vi "Biometry Average PD Parameter2String.vi"(8 "error in (no error)":errorcluster caption="错误输入（无错误）", 9 "Biometry Average Standard Deviation":T1, 10 "Biometry Average State":T2, 11 "Biometry Average Parameter":T3) -> (0 "error out":errorcluster caption="错误输出", 2 "Data Output":string[][](array[string]))   [LabVIEW 2015, in "Utility VIs.lvlib"]
doc: "该模板用于创建子VI。"
uses:
  Utility VIs.lvlib
  Database Processing/Support/Table/Biometry Average Parameter.ctl
  Database Processing/Support/Table/Biometry Average State.ctl
  Database Processing/Support/Table/Biometry Average Standard Deviation.ctl
  Database Processing/Database Processing.lvlib
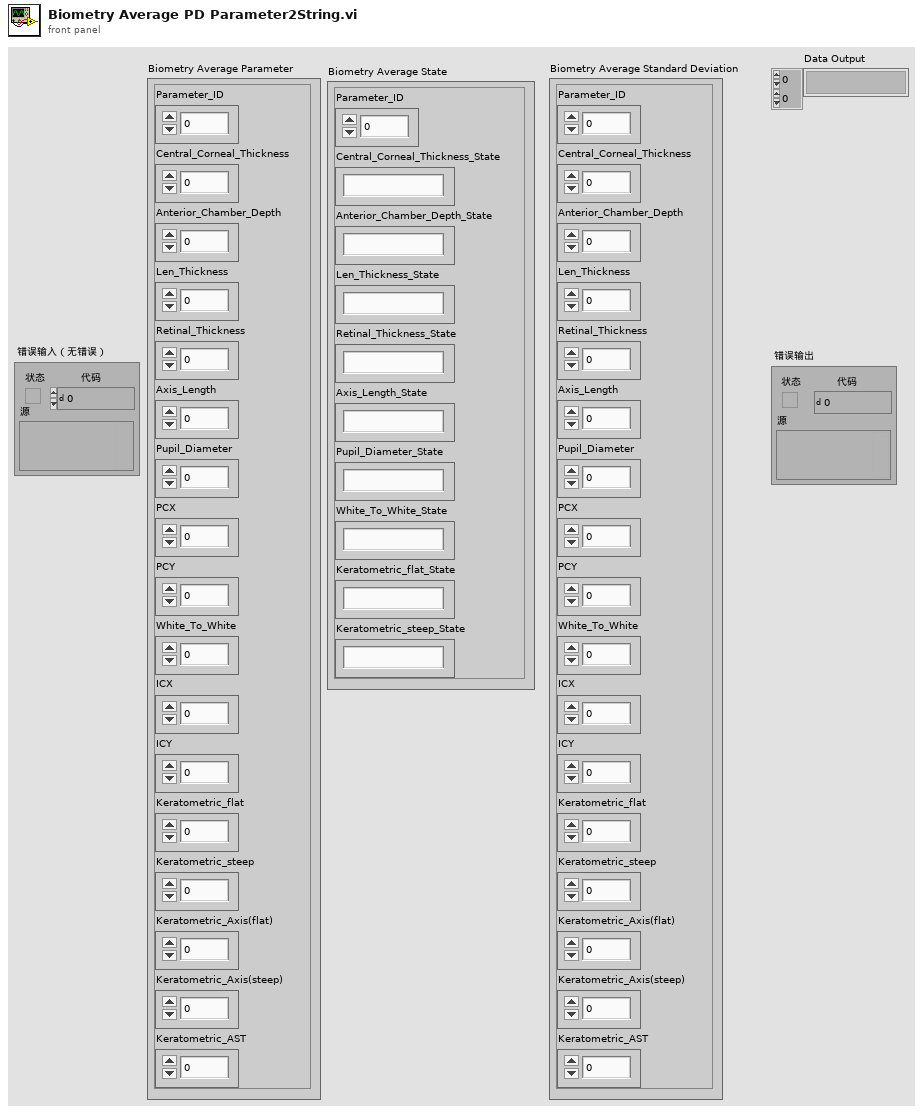
[diagram p1: front panel]
types:
  T1 = typedef "Database Processing.lvlib/Biometry Average Standard Deviation.ctl" = cluster{"Parameter_ID":i64, "Central_Corneal_Thickness":sgl, "Anterior_Chamber_Depth":sgl, "Len_Thickness":sgl, "Retinal_Thickness":sgl, "Axis_Length":sgl, "Pupil_Diameter":sgl, "PCX":sgl, "PCY":sgl, "White_To_White":sgl, "ICX":sgl, "ICY":sgl, "Keratometric_flat":sgl, "Keratometric_steep":sgl, "Keratometric_Axis(flat)":sgl, "Keratometric_Axis(steep)":sgl, "Keratometric_AST":sgl}
  T2 = typedef "Database Processing.lvlib/Biometry Average State.ctl" = cluster{"Parameter_ID":i64, "Central_Corneal_Thickness_State":string, "Anterior_Chamber_Depth_State":string, "Len_Thickness_State":string, "Retinal_Thickness_State":string, "Axis_Length_State":string, "Pupil_Diameter_State":string, "White_To_White_State":string, "Keratometric_flat_State":string, "Keratometric_steep_State":string}
  T3 = typedef "Database Processing.lvlib/Biometry Average Parameter.ctl" = cluster{"Parameter_ID":i64, "Central_Corneal_Thickness":sgl, "Anterior_Chamber_Depth":sgl, "Len_Thickness":sgl, "Retinal_Thickness":sgl, "Axis_Length":sgl, "Pupil_Diameter":sgl, "PCX":sgl, "PCY":sgl, "White_To_White":sgl, "ICX":sgl, "ICY":sgl, "Keratometric_flat":sgl, "Keratometric_steep":sgl, "Keratometric_Axis(flat)":sgl, "Keratometric_Axis(steep)":sgl, "Keratometric_AST":sgl}
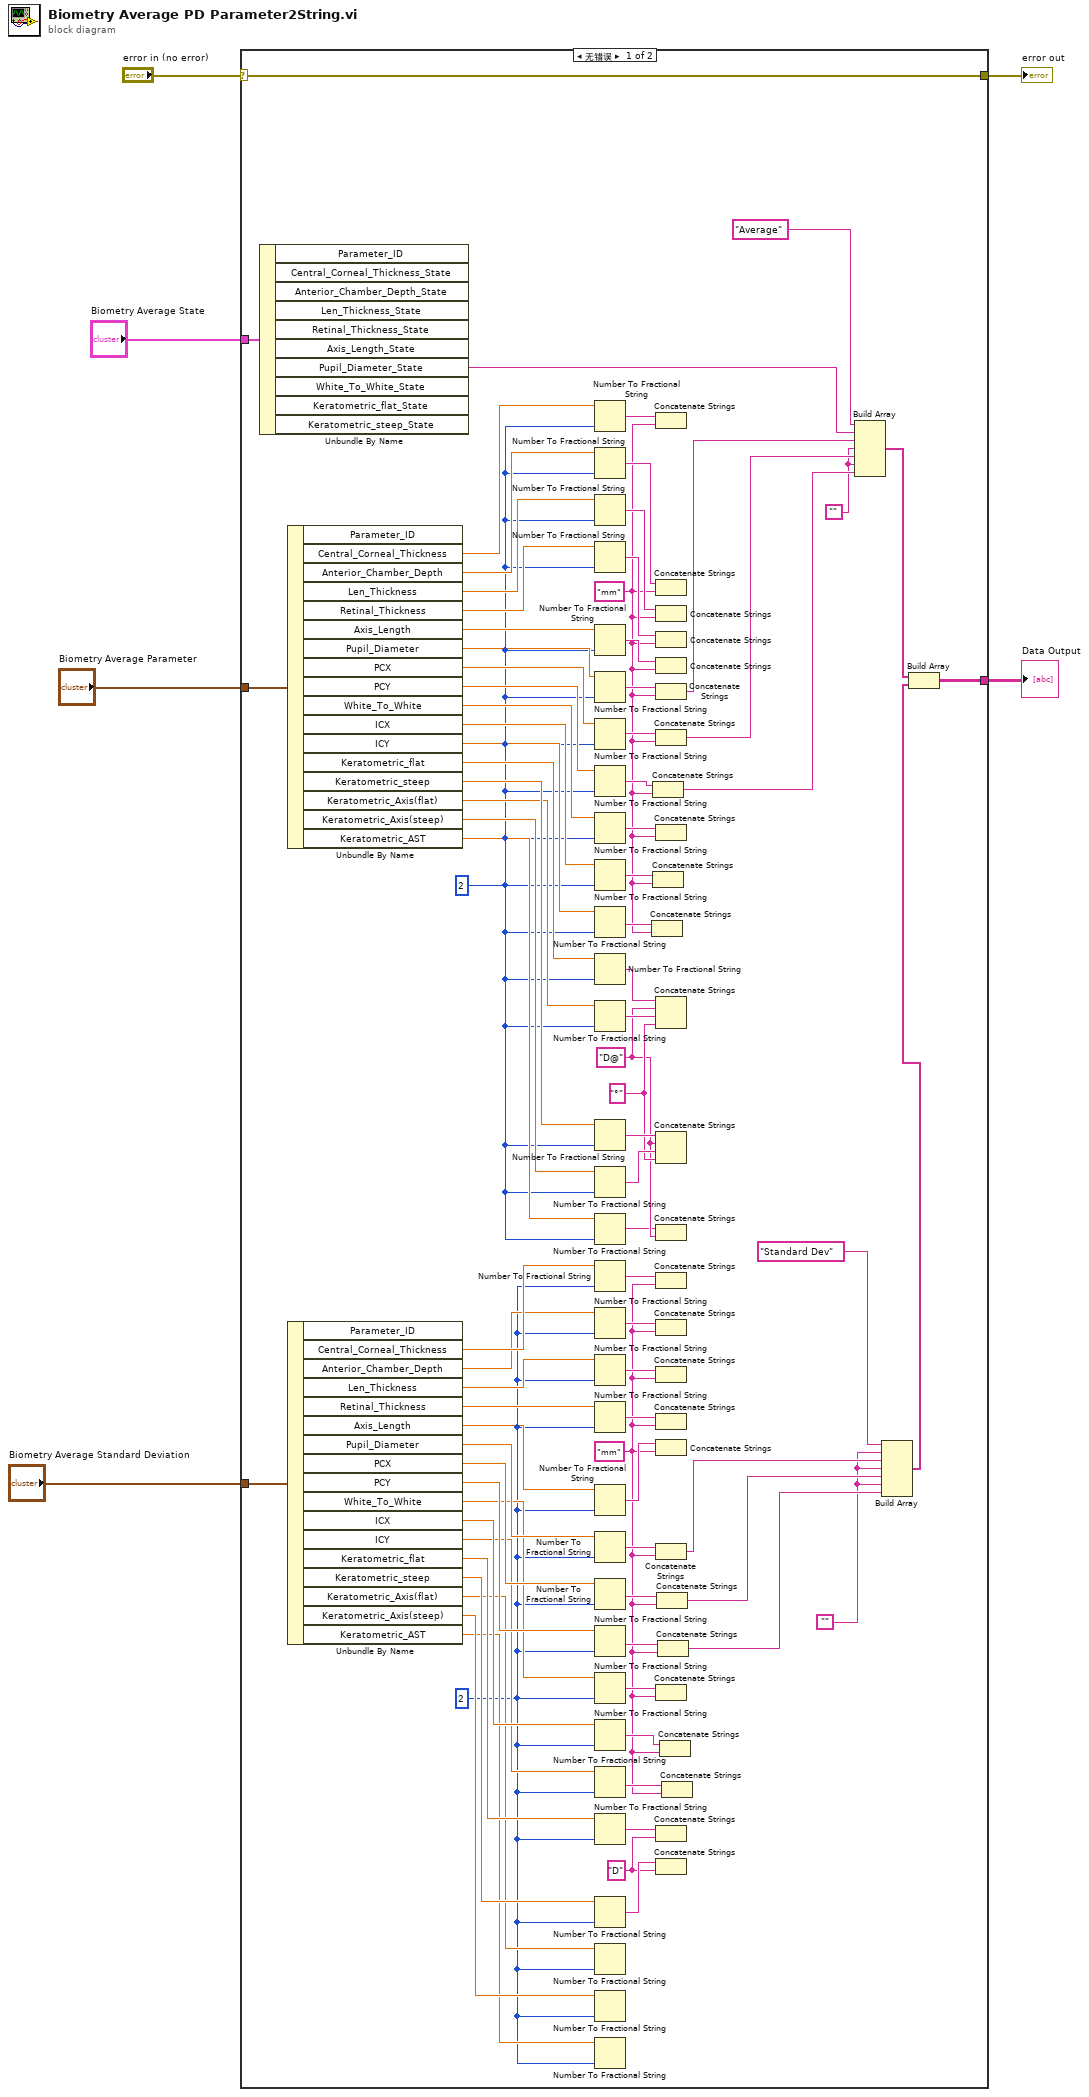
[diagram p0: block diagram]
diagram:
  n1 = case shown="无错误" "error in (no error)" {
    selector: "error in (no error)" -> [w33 w93]
    tunnel: [w33 w93] -> w5
    tunnel: "Biometry Average Parameter" -> [w92 _]
    tunnel: "Biometry Average Standard Deviation" -> [w91 _]
    tunnel: "Biometry Average State" -> [w90 _]
    tunnel: [w17 _] -> w1
    frame No Error {
      w11 = ""
      w7 = ""
      w34 = "D" ("字符串")
      w21 = "mm" ("字符串")
      w37 = i16 2 ("精度(6)")
      w47 = "°" ("字符串")
      w27 = "D@" ("字符串")
      w28 = "mm" ("字符串")
      w49 = i16 2 ("精度(6)")
      n2 = Unbundle By Name(w90) -> ("Pupil_Diameter_State"=w15:string)  [unwired: 9 out]
      n3 = Unbundle By Name(w92) -> ("Central_Corneal_Thickness"=w89:sgl, "Anterior_Chamber_Depth"=w88:sgl, "Len_Thickness"=w87:sgl, "Retinal_Thickness"=w86:sgl, "Axis_Length"=w85:sgl, "Pupil_Diameter"=w84:sgl, "PCX"=w83:sgl, "PCY"=w82:sgl, "White_To_White"=w81:sgl, "ICX"=w80:sgl, "ICY"=w79:sgl, "Keratometric_flat"=w78:sgl, "Keratometric_steep"=w77:sgl, "Keratometric_Axis(flat)"=w76:sgl, "Keratometric_Axis(steep)"=w51:sgl, "Keratometric_AST"=w50:sgl)  [unwired: 1 out]
      n4 = Unbundle By Name(w91) -> ("Central_Corneal_Thickness"=w75:sgl, "Anterior_Chamber_Depth"=w74:sgl, "Len_Thickness"=w73:sgl, "Retinal_Thickness"=w72:sgl, "Axis_Length"=w71:sgl, "Pupil_Diameter"=w70:sgl, "PCX"=w69:sgl, "PCY"=w68:sgl, "White_To_White"=w67:sgl, "ICX"=w66:sgl, "ICY"=w65:sgl, "Keratometric_flat"=w64:sgl, "Keratometric_steep"=w63:sgl, "Keratometric_Axis(flat)"=w62:sgl, "Keratometric_Axis(steep)"=w39:sgl, "Keratometric_AST"=w38:sgl)  [unwired: 1 out]
      n5 = Number To Fractional String(number=w89, precision (6)=w49) -> (F-format string=w61:string)  [unwired: 2 in]
      n6 = Number To Fractional String(number=w88, precision (6)=w49) -> (F-format string=w60:string)  [unwired: 2 in]
      n7 = Number To Fractional String(number=w87, precision (6)=w49) -> (F-format string=w59:string)  [unwired: 2 in]
      n8 = Number To Fractional String(number=w86, precision (6)=w49) -> (F-format string=w58:string)  [unwired: 2 in]
      n9 = Number To Fractional String(number=w85, precision (6)=w49) -> (F-format string=w57:string)  [unwired: 2 in]
      n10 = Number To Fractional String(number=w84, precision (6)=w49) -> (F-format string=w56:string)  [unwired: 2 in]
      n11 = Number To Fractional String(number=w83, precision (6)=w49) -> (F-format string=w32:string)  [unwired: 2 in]
      n12 = Number To Fractional String(number=w82, precision (6)=w49) -> (F-format string=w31:string)  [unwired: 2 in]
      n13 = Number To Fractional String(number=w81, precision (6)=w49) -> (F-format string=w55:string)  [unwired: 2 in]
      n14 = Number To Fractional String(number=w80, precision (6)=w49) -> (F-format string=w30:string)  [unwired: 2 in]
      n15 = Number To Fractional String(number=w79, precision (6)=w49) -> (F-format string=w29:string)  [unwired: 2 in]
      n16 = Number To Fractional String(number=w78, precision (6)=w49) -> (F-format string=w54:string)  [unwired: 2 in]
      n17 = Number To Fractional String(number=w76, precision (6)=w49) -> (F-format string=w52:string)  [unwired: 2 in]
      n18 = Number To Fractional String(number=w77, precision (6)=w49) -> (F-format string=w53:string)  [unwired: 2 in]
      n19 = Number To Fractional String(number=w51, precision (6)=w49) -> (F-format string=w48:string)  [unwired: 2 in]
      n20 = Number To Fractional String(number=w50, precision (6)=w49) -> (F-format string=w26:string)  [unwired: 2 in]
      n21 = Number To Fractional String(number=w75, precision (6)=w37) -> (F-format string=w46:string)  [unwired: 2 in]
      n22 = Number To Fractional String(number=w74, precision (6)=w37) -> (F-format string=w45:string)  [unwired: 2 in]
      n23 = Number To Fractional String(number=w73, precision (6)=w37) -> (F-format string=w44:string)  [unwired: 2 in]
      n24 = Number To Fractional String(number=w72, precision (6)=w37) -> (F-format string=w43:string)  [unwired: 2 in]
      n25 = Number To Fractional String(number=w71, precision (6)=w37) -> (F-format string=w42:string)  [unwired: 2 in]
      n26 = Number To Fractional String(number=w70, precision (6)=w37) -> (F-format string=w41:string)  [unwired: 2 in]
      n27 = Number To Fractional String(number=w69, precision (6)=w37) -> (F-format string=w25:string)  [unwired: 2 in]
      n28 = Number To Fractional String(number=w68, precision (6)=w37) -> (F-format string=w24:string)  [unwired: 2 in]
      n29 = Number To Fractional String(number=w67, precision (6)=w37) -> (F-format string=w40:string)  [unwired: 2 in]
      n30 = Number To Fractional String(number=w66, precision (6)=w37) -> (F-format string=w23:string)  [unwired: 2 in]
      n31 = Number To Fractional String(number=w65, precision (6)=w37) -> (F-format string=w22:string)  [unwired: 2 in]
      n32 = Number To Fractional String(number=w64, precision (6)=w37) -> (F-format string=w36:string)  [unwired: 2 in]
      n33 = Number To Fractional String(number=w63, precision (6)=w37) -> (F-format string=w35:string)  [unwired: 2 in]
      n34 = Number To Fractional String(number=w62, precision (6)=w37) -> ()  [unwired: 2 in, 1 out]
      n35 = Number To Fractional String(number=w39, precision (6)=w37) -> ()  [unwired: 2 in, 1 out]
      n36 = Number To Fractional String(number=w38, precision (6)=w37) -> ()  [unwired: 2 in, 1 out]
      n37 = Concatenate Strings(w29, w28) -> ()  [unwired: 1 out]
      n38 = Concatenate Strings(w31, w28) -> (w12:string)
      n39 = Concatenate Strings(w30, w28) -> ()  [unwired: 1 out]
      n40 = Concatenate Strings(w61, w28) -> ()  [unwired: 1 out]
      n41 = Concatenate Strings(w60, w28) -> ()  [unwired: 1 out]
      n42 = Concatenate Strings(w59, w28) -> ()  [unwired: 1 out]
      n43 = Concatenate Strings(w58, w28) -> ()  [unwired: 1 out]
      n44 = Concatenate Strings(w57, w28) -> ()  [unwired: 1 out]
      n45 = Concatenate Strings(w56, w28) -> (w14:string)
      n46 = Concatenate Strings(w32, w28) -> (w13:string)
      n47 = Concatenate Strings(w55, w28) -> ()  [unwired: 1 out]
      n48 = Concatenate Strings(w54, w27, w52, w47) -> ()  [unwired: 1 out]
      n49 = Concatenate Strings(w53, w27, w48, w47) -> ()  [unwired: 1 out]
      n50 = Concatenate Strings(w26, w27) -> ()  [unwired: 1 out]
      n51 = Concatenate Strings(w46, w21) -> ()  [unwired: 1 out]
      n52 = Concatenate Strings(w45, w21) -> ()  [unwired: 1 out]
      n53 = Concatenate Strings(w44, w21) -> ()  [unwired: 1 out]
      n54 = Concatenate Strings(w43, w21) -> ()  [unwired: 1 out]
      n55 = Concatenate Strings(w42, w21) -> ()  [unwired: 1 out]
      n56 = Concatenate Strings(w41, w21) -> (w10:string)
      n57 = Concatenate Strings(w40, w21) -> ()  [unwired: 1 out]
      n58 = Concatenate Strings(w36, w34) -> ()  [unwired: 1 out]
      n59 = Concatenate Strings(w35, w34) -> ()  [unwired: 1 out]
      n60 = Concatenate Strings(w25, w21) -> (w9:string)
      n61 = Concatenate Strings(w24, w21) -> (w8:string)
      n62 = Concatenate Strings(w23, w21) -> ()  [unwired: 1 out]
      n63 = Concatenate Strings(w22, w21) -> ()  [unwired: 1 out]
      n64 = Build Array("Average" ("元素"), w15, w14, w11, w13, w11, w12) -> (w19:string[])
      n65 = Build Array("Standard Dev" ("元素"), w7, w10, w7, w9, w7, w8) -> (w18:string[])
      n66 = Build Array(w19, w18) -> (w17:string[][])
    }
    frame Error {
    }
  }
  "error out" <- w5
  "Data Output" <- w1
